vi "temperatura (SubVI).vi"(11 "data in":string) -> (3 "Numeric":dbl)   [LabVIEW 2015]
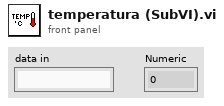
[diagram p1: front panel]
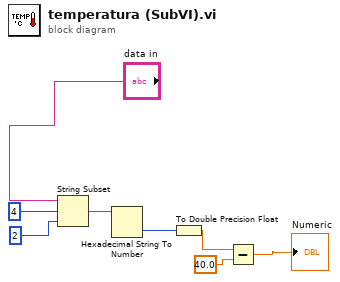
[diagram p0: block diagram]
diagram:
  n1 = String Subset(string="data in", offset (0)=4, length (rest)=2 ("length (rest)")) -> (substring=w6:string)
  n2 = Hexadecimal String To Number(string=w6) -> (number=w5:u32)  [unwired: 2 in, 1 out]
  n3 = To Double Precision Float(number=w5) -> (double precision float=w2:dbl)
  n4 = Subtract(x=w2, y=40.0) -> (x-y=→"Numeric":dbl)
